vi "JKISM++ Convert Argument to Array.vi"(2 "HEX Argument":string) -> (7 "DBL":dbl[](array[numeric]))   [LabVIEW 2020, in "JKISM++ Array Parameter Support.lvlib"]
doc: "Convert hex string arguments back to variant.\n\n<b>Inputs:</b>\n - <b>HEX String</b>: Hex String, which contains no invisible string following JKISM's rule\n\n<b>Outputs:</b>\n - <b>Variant</b>: Complex data in variant format."
uses:
  JKISM++ Array Parameter Support.lvlib
  _support/Operation-FGV-MassData.ctl
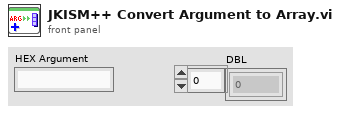
[diagram p1: front panel]
types:
  T1 = typedef "JKISM++ Array Parameter Support.lvlib/Operation-FGV-MassData.ctl" = enum16{"Initialize", "Read", "Write", "Status", "Release"}
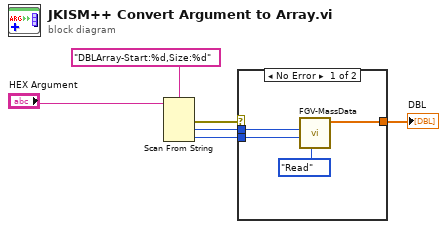
[diagram p0: block diagram]
diagram:
  n1 = Scan From String(format string="DBLArray-Start:%d,Size:%d", input string="HEX Argument") -> (error out=w1:errorcluster, output 1=w4:i32, output 2=w3:i32)  [unwired: 4 in, 2 out]
  n2 = case shown="No Error" w1 {
    tunnel: w4 -> [w9 _]
    tunnel: w3 -> [w8 _]
    tunnel: [w7 _] -> w2
    frame No Error {
      n3 = call "FGV-MassData.vi"("Operation"=Operation-FGV-MassData."Read", "size"=w8, "Start"=w9) -> ("Data out"=w7:dbl[])  [unwired: 5 in, 3 out]
    }
    frame Error {
    }
  }
  "DBL" <- w2
